vi "Debugging RT Channels.vi"(5 "Output FIFO Length":i32, 7 "Input FIFO Length":i32, 8 "Output FIFO Index":i32, 9 "Input FIFO Index":i32, 10 "Output  Channel Refs":T1[](array[typedef]) format="%.0x", 11 "Input Channel Refs":T1[](array[typedef]) format="%.0x") -> ()   [LabVIEW 2019, in "SEECD Engine.lvlib"]
uses:
  SEECD Engine.lvlib
  <vilib>/NI VeriStand/Custom Device Tools/Custom Device Utility Library/Custom Device Utility Library.lvlib
  Shared/Globals/Property Strings.vi
  Shared/SEECD Shared.lvlib
  <vilib>/NI VeriStand/Custom Device API/Custom Device API.lvlib
  <vilib>/NI VeriStand/Custom Device API/Custom Device Item Ref.ctl
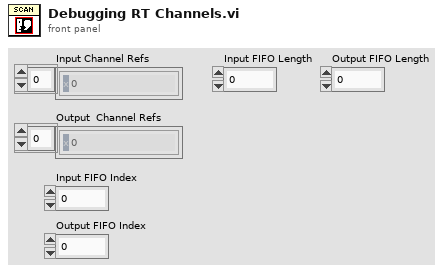
[diagram p1: front panel]
types:
  T1 = typedef "Custom Device API.lvlib/Custom Device Item Ref.ctl" = u64
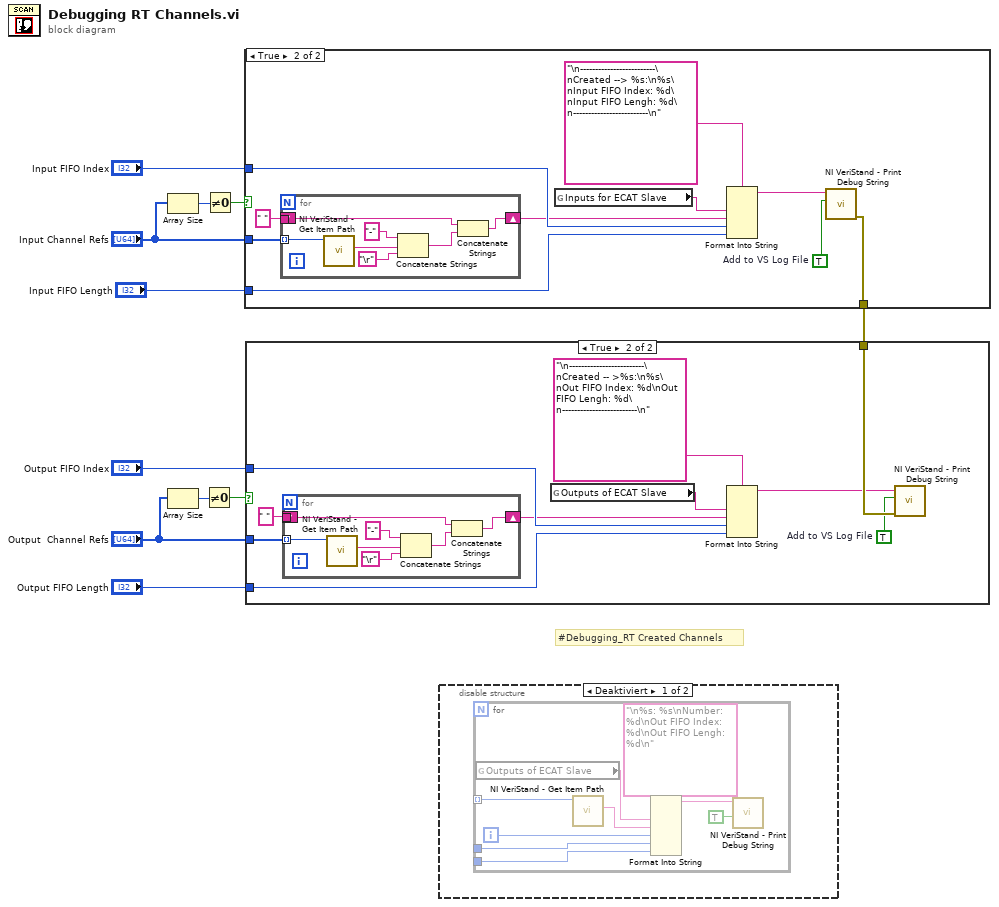
[diagram p0: block diagram]
diagram:
  # "#Debugging_RT Created Channels"
  n1 = Array Size(array="Input Channel Refs") -> (size(s)=w5:i32)
  n2 = Array Size(array="Output  Channel Refs") -> (size(s)=w3:i32)
  n3 = Not Equal To 0?(x=w3) -> (x != 0?=w2:bool)
  n4 = Not Equal To 0?(x=w5) -> (x != 0?=w6:bool)
  n5 = case shown="True" w6 {
    tunnel: "Input FIFO Length" -> [_ w21]
    tunnel: "Input FIFO Index" -> [_ w20]
    tunnel: "Input Channel Refs" -> [_ w18]
    tunnel: [_ w15] -> w7
    frame False {
    }
    frame True {
      w13 = TRUE  # Add to VS Log File
      w17 = " "
      n6 = for {
        tunnel: w17 -> [_]
        shift-right: [w23] -> w14
        shift-left: w17 -> [w24]
        tunnel: w18 -> [w25] mode=indexing
        n7 = call <vilib>:"NI VeriStand - Get Item Path.vi"("Item Ref in"=w25) -> ("Path"=w26:string)  [unwired: 7 in, 3 out]
        n8 = Concatenate Strings("-", w26, "\r") -> (w22:string)
        n9 = Concatenate Strings(w24, w22) -> (w23:string)
      }
      n10 = global read "Property Strings.vi" "Inputs for ECAT Slave"() -> (w16:string)
      n11 = Format Into String(format string="\n-------------------------\nCreated --> %s:\n%s\nInput FIFO Index: %d\nInput FIFO Lengh: %d\n-------------------------\n" ("Format-String"), w16, w14, w20, w21) -> (resulting string=w12:string)  [unwired: 2 in, 1 out]
      n12 = call <vilib>:"NI VeriStand - Print Debug String.vi"("Add to log file? (F)"=w13, "Message"=w12) -> ("error out"=w15:errorcluster)  [unwired: 9 in]
    }
  }
  n13 = case shown="True" w2 {
    tunnel: "Output FIFO Length" -> [_ w38]
    tunnel: "Output FIFO Index" -> [_ w37]
    tunnel: "Output  Channel Refs" -> [_ w36]
    tunnel: w7 -> [_ w32]
    frame False {
    }
    frame True {
      w30 = TRUE  # Add to VS Log File
      w35 = " "
      n14 = for {
        tunnel: w35 -> [_]
        shift-right: [w41] -> w31
        shift-left: w35 -> [w40]
        tunnel: w36 -> [w42] mode=indexing
        n15 = call <vilib>:"NI VeriStand - Get Item Path.vi"("Item Ref in"=w42) -> ("Path"=w43:string)  [unwired: 7 in, 3 out]
        n16 = Concatenate Strings("-", w43, "\r") -> (w39:string)
        n17 = Concatenate Strings(w40, w39) -> (w41:string)
      }
      n18 = global read "Property Strings.vi" "Outputs of ECAT Slave"() -> (w33:string)
      n19 = Format Into String(format string="\n-------------------------\nCreated -- >%s:\n%s\nOut FIFO Index: %d\nOut FIFO Lengh: %d\n-------------------------\n" ("Format-String"), w33, w31, w37, w38) -> (resulting string=w29:string)  [unwired: 2 in, 1 out]
      n20 = call <vilib>:"NI VeriStand - Print Debug String.vi"("error in (no error)"=w32, "Add to log file? (F)"=w30, "Message"=w29) -> ()  [unwired: 8 in, 1 out]
    }
  }
  n21 = disable-structure shown="Deaktiviert" {
    frame Disabled {
      n22 = for {
        tunnel: _ -> [w54] mode=indexing
        tunnel: _ -> [w46]
        tunnel: _ -> [w47]
        i -> [w52]
        n23 = global read "Property Strings.vi" "Outputs of ECAT Slave"() -> (w50:string)
        n24 = call <vilib>:"NI VeriStand - Get Item Path.vi"("Item Ref in"=w54) -> ("Path"=w49:string)  [unwired: 7 in, 3 out]
        n25 = Format Into String(format string="\n%s: %s\nNumber: %d\nOut FIFO Index: %d\nOut FIFO Lengh: %d\n" ("Format-String"), w50, w49, w52, w46, w47) -> (resulting string=w51:string)  [unwired: 2 in, 1 out]
        n26 = call <vilib>:"NI VeriStand - Print Debug String.vi"("Add to log file? (F)"=TRUE, "Message"=w51) -> ()  [unwired: 9 in, 1 out]
      }
    }
    frame Enabled {
    }
  }
